vi "MCP2221_Output_Sample.vi"() -> ()   [LabVIEW 2025]
panel:
  out "error out":errorcluster
  in  "stop":bool
  in  "GP3":bool
  in  "GP2":bool
  in  "GP1":bool
  in  "GP0":bool
  # "ON"
  # "OFF"
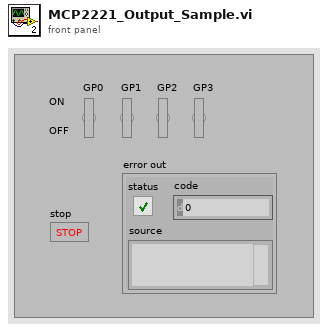
[diagram p1: front panel]
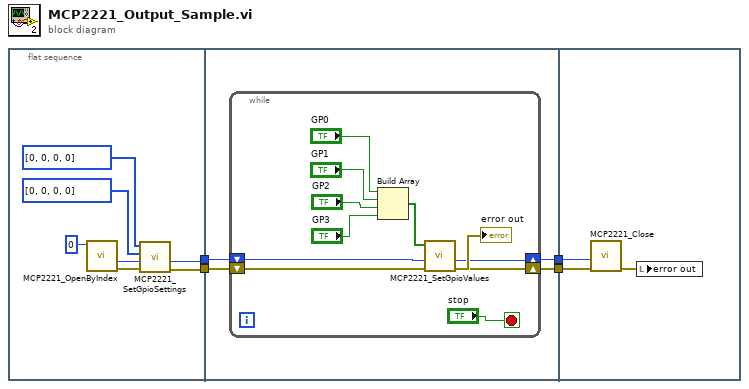
[diagram p0: block diagram]
diagram:
  n1 = flat-sequence {
    tunnel: [w8] -> w4
    tunnel: [w7] -> w3
    tunnel: w4 -> [w15]
    tunnel: w3 -> [w14]
    tunnel: [w13] -> w2
    tunnel: [w12] -> w1
    tunnel: w2 -> [w28]
    tunnel: w1 -> [w27]
    frame #0 {
      n2 = call "MCP2221_OpenByIndex.vi"("index"=u32 0) -> ("error out"=w10:errorcluster, "handle out"=w9:i32)  [unwired: 9 in]
      n3 = call "MCP2221_SetGpioSettings.vi"("error in"=w10, "handle in"=w9, "outputValues"=u8[] [0, 0, 0, 0] ("pinDirections"), "pinDirections"=u8[] [0, 0, 0, 0]) -> ("error out"=w8:errorcluster, "handle out"=w7:i32)  [unwired: 5 in, 1 out]
    }
    frame #1 {
      n4 = while {
        shift-right: [w21] -> w12
        shift-left: w14 -> [w25]
        shift-right: [w22] -> w13
        shift-left: w15 -> [w24]
        stop <- "stop" stop-if-true
        n5 = Build Array("GP0", "GP1", "GP2", "GP3") -> (w23:bool[])
        n6 = call "MCP2221_SetGpioValues.vi"("error in"=w24, "handle in"=w25, "gpio"=w23) -> ("error out"=w22:errorcluster, "handle out"=w21:i32)  [unwired: 6 in, 1 out]
        "error out" <- w24
      }
    }
    frame #2 {
      n7 = call "MCP2221_Close.vi"("error in"=w28, "handle in"=w27) -> ("error out"=w26:errorcluster)  [unwired: 7 in, 2 out]
      n8 = local write "error out"(w26) -> ()
    }
  }
